vi "SolarPanel_Analysis_v0.4-1.vi"() -> ()   [LabVIEW 2021]
uses:
  <vilib>/Utility/file.llb/Write Delimited Spreadsheet (DBL).vi
  <vilib>/Utility/file.llb/Write Delimited Spreadsheet (string).vi
  <vilib>/express/express arith-compare/Formula/XNode/ExpressFormulaBlockNode.xnode
  <vilib>/Analysis/NI_AALBase.lvlib
panel:
  in  "R":dbl
  out "Experiment Power [W]":dbl format="%_6g"
  out "Control Power [W]":dbl format="%_6g"
  in  "device name":tag="Dev1"
  out "Experiment Power":waveform(dbl)(graph)
  out "Experiment Panel Voltage [V]":dbl format="%_6g"
  in  "file path (dialog if empty)":path
  in  "Number of Samples":i32=100
  in  "Sampling Rate [Hz]":dbl=1000.0
  out "Control Power":waveform(dbl)(graph)
  in  "?":bool
  in  "Format (%.6f)":string="%.6f"
  out "Time [s]":dbl
  out "Control Panel Voltage [V]":dbl format="%_6g"
  out "Servo Voltage [V]":dbl format="%_6g"
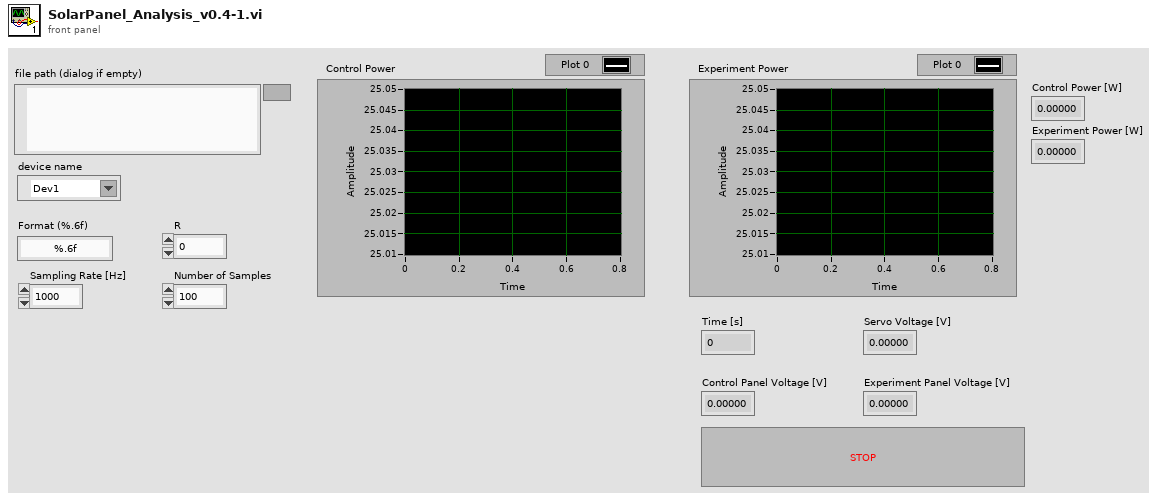
[diagram p1: front panel]
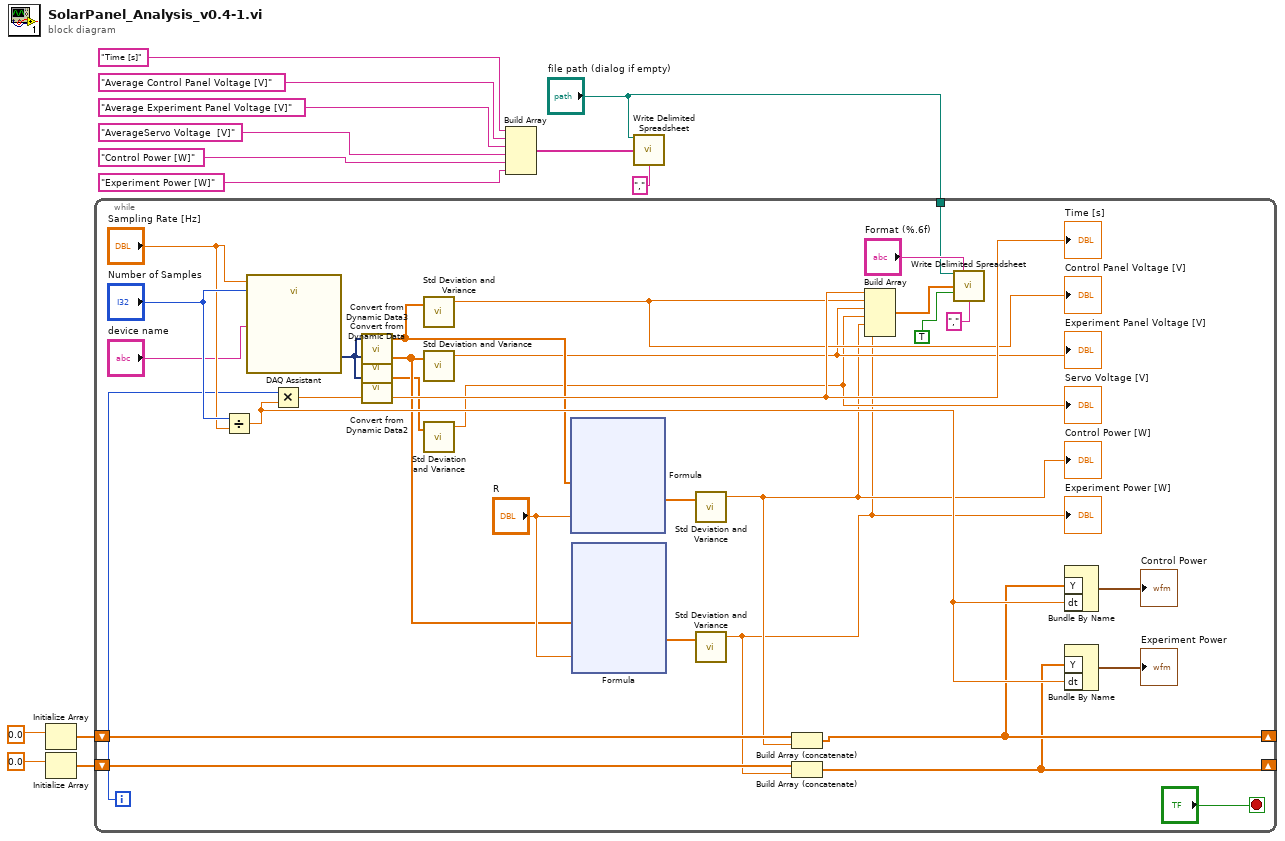
[diagram p0: block diagram]
diagram:
  n1 = Initialize Array(0.0) -> (w6:dbl[])  [unwired: 1 in]
  n2 = Initialize Array(0.0) -> (w3:dbl[])  [unwired: 1 in]
  n3 = while {
    tunnel: "file path (dialog if empty)" -> [w33]
    shift-right: [w24] -> _
    shift-left: w6 -> [w32]
    shift-right: [w23] -> _
    shift-left: w3 -> [w30]
    i -> [w38]
    stop <- "?" stop-if-true
    n4 = Divide(x="Number of Samples", y="Sampling Rate [Hz]") -> (x/y=w29:dbl)
    n5 = call "DAQ Assistant"("rate"="Sampling Rate [Hz]", "number of samples"="Number of Samples", "device name"="device name") -> ("data"=w22:dynamicdata)  [unwired: 14 in, 2 out]
    n6 = Multiply(x=w38, y=w29) -> (x*y=w34:dbl)
    "Time [s]" <- w34
    n7 = call "Convert from Dynamic Data3"("Dynamic Data Type"=w22) -> ("Array"=w19:dbl[])  [unwired: 3 in]
    n8 = call "Convert from Dynamic Data"("Dynamic Data Type"=w22) -> ("Array"=w21:dbl[])  [unwired: 3 in]
    n9 = call "Convert from Dynamic Data2"("Dynamic Data Type"=w22) -> ("Array"=w20:dbl[])  [unwired: 3 in]
    n10 = call <vilib>:"Std Deviation and Variance.vi"("X"=w19) -> ("mean"=w18:dbl)  [unwired: 1 in, 2 out]
    "Control Panel Voltage [V]" <- w18
    n11 = call <vilib>:"Std Deviation and Variance.vi"("X"=w21) -> ("mean"=w17:dbl)  [unwired: 1 in, 2 out]
    "Experiment Panel Voltage [V]" <- w17
    n12 = call <vilib>:"Std Deviation and Variance.vi"("X"=w20) -> ("mean"=w16:dbl)  [unwired: 1 in, 2 out]
    "Servo Voltage [V]" <- w16
    n13 = xnode "Formula"("V"=w19, "R"="R") -> ("Result"=w26:dbl[])  [unwired: 1 in, 1 out]
    n14 = xnode "Formula"("Vp"=w21, "R"="R") -> ("Result"=w25:dbl[])  [unwired: 1 in, 1 out]
    n15 = call <vilib>:"Std Deviation and Variance.vi"("X"=w26) -> ("mean"=w15:dbl)  [unwired: 1 in, 2 out]
    "Control Power [W]" <- w15
    n16 = call <vilib>:"Std Deviation and Variance.vi"("X"=w25) -> ("mean"=w14:dbl)  [unwired: 1 in, 2 out]
    "Experiment Power [W]" <- w14
    n17 = Build Array (concatenate)(w32, w15) -> (w24:dbl[])
    n18 = Build Array (concatenate)(w30, w14) -> (w23:dbl[])
    n19 = Build Array(w34, w18, w17, w16, w15, w14) -> (w42:dbl[])
    n20 = call-poly <vilib>:"Write Delimited Spreadsheet.vi"("file path (dialog if empty)"=w33, "format (%.3f)"="Format (%.6f)", "1D data"=w42, "append to file? (new file:F)"=TRUE, "delimiter (\\t)"=",") -> ()  [unwired: 9 in, 2 out]
    n21 = Bundle By Name("Y"=w24, "dt"=w29) -> (→"Control Power":waveform(dbl))  [unwired: 1 in]
    n22 = Bundle By Name("Y"=w23, "dt"=w29) -> (→"Experiment Power":waveform(dbl))  [unwired: 1 in]
  }
  n23 = Build Array("Time [s]", "Average Control Panel Voltage [V]", "Average Experiment Panel Voltage [V]", "AverageServo Voltage  [V]", "Control Power [W]", "Experiment Power [W]") -> (w13:string[])
  n24 = call-poly <vilib>:"Write Delimited Spreadsheet.vi"("file path (dialog if empty)"="file path (dialog if empty)", "1D data"=w13, "delimiter (\\t)"=",") -> ()  [unwired: 11 in, 2 out]
